vi "Create_zero_waveform.vi"(11 "Waveform in":waveform(cdb)) -> (3 "Waveform out":waveform(cdb))   [LabVIEW 2018]
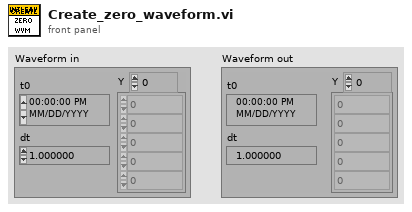
[diagram p1: front panel]
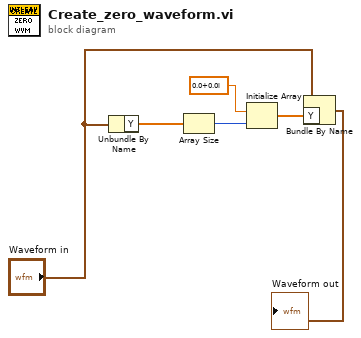
[diagram p0: block diagram]
diagram:
  n1 = Unbundle By Name("Waveform in") -> ("Y"=w1:cdb[])
  n2 = Array Size(array=w1) -> (size(s)=w2:i32)
  n3 = Initialize Array(cdb 0.0+0.0i ("element"), w2) -> (w4:cdb[])
  n4 = Bundle By Name(cluster="Waveform in", "Y"=w4) -> (→"Waveform out":waveform(cdb))
